vi "setTime.vi"(0 "connection ID":refnum<k5>, 1 "day":i32, 2 "month":i32, 3 "year":i32, 4 "hour":i32, 5 "error":errorcluster, 6 "minute":i32, 7 "second":i32) -> (14 "connection ID out":refnum<k5>, 19 "error out":errorcluster)   [LabVIEW 2016, in "amc_api.lvlib"]
doc: "Sets system time manually."
uses:
  amc_api.lvlib
panel:
  out "jsonRespIn":string
  out "JSON-response":string="{\"jsonrpc\":\"2.0\",\"method\":\"\",\"params\":[5,1.245,true,\"name\"],\"id\":\"1\"}"
  out "JSON request":string
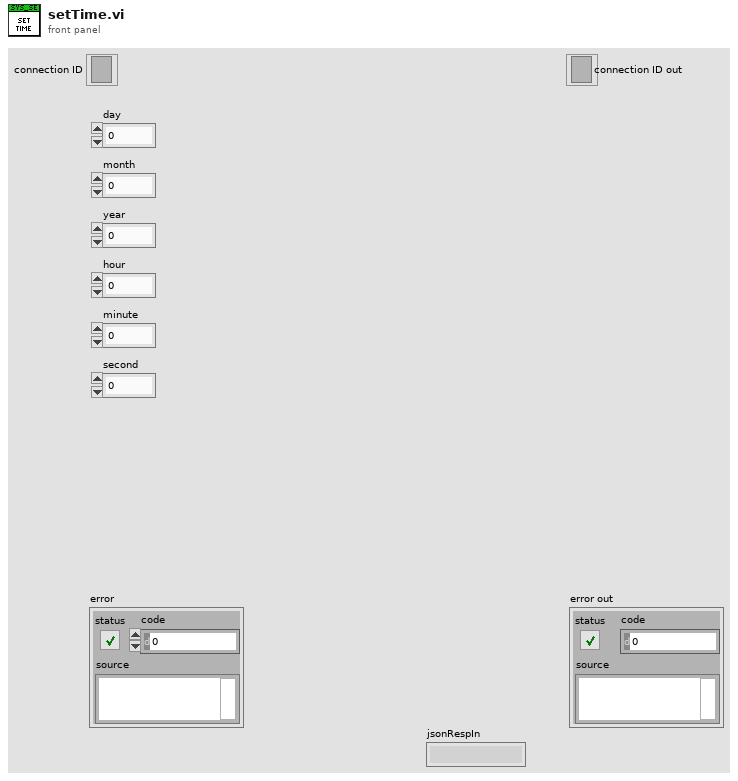
[diagram p1: front panel]
types:
  T1 = cluster{"jsonrpc":string, "method":string, "params":string[], "id":string, "api":i32, "pid":string}
  T2 = enum16{"Standard", "Buffered", "CRLF", "Immediate"}
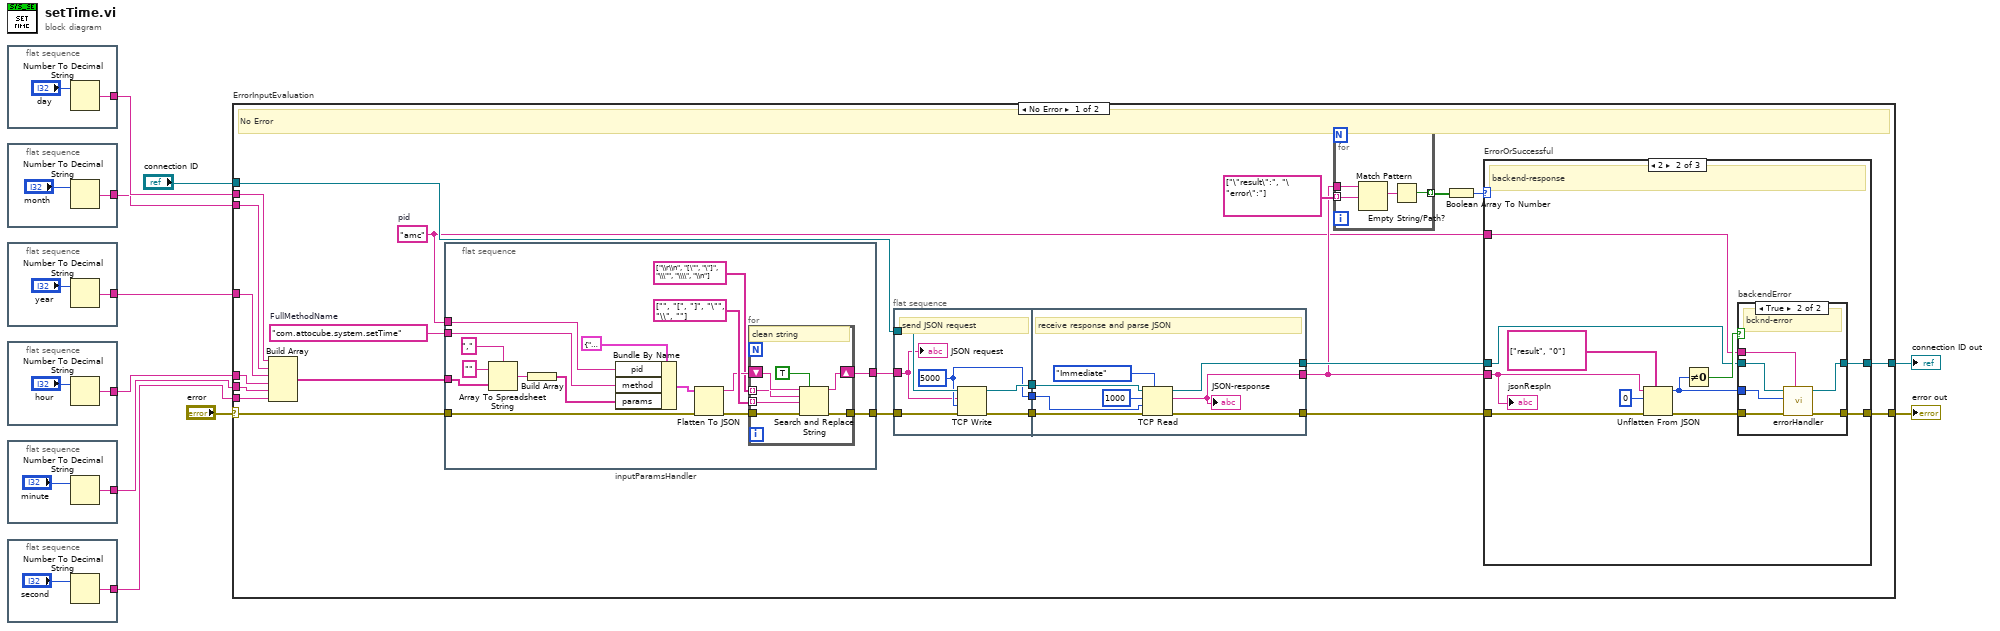
[diagram p0: block diagram]
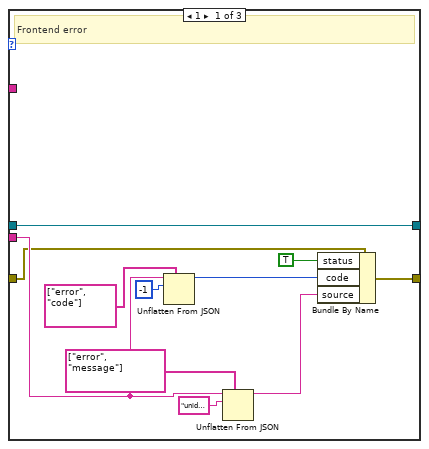
[diagram p2: hidden frame]
diagram:
  n1 = flat-sequence "in_integer" {
    tunnel: [w11] -> w6
    frame #0 {
      n2 = Number To Decimal String(number="day") -> (decimal integer string=w11:string)  [unwired: 1 in]
    }
  }
  n3 = flat-sequence "in_integer" {
    tunnel: [w13] -> w5
    frame #0 {
      n4 = Number To Decimal String(number="month") -> (decimal integer string=w13:string)  [unwired: 1 in]
    }
  }
  n5 = flat-sequence "in_integer" {
    tunnel: [w15] -> w4
    frame #0 {
      n6 = Number To Decimal String(number="year") -> (decimal integer string=w15:string)  [unwired: 1 in]
    }
  }
  n7 = flat-sequence "in_integer" {
    tunnel: [w17] -> w3
    frame #0 {
      n8 = Number To Decimal String(number="hour") -> (decimal integer string=w17:string)  [unwired: 1 in]
    }
  }
  n9 = flat-sequence "in_integer" {
    tunnel: [w19] -> w2
    frame #0 {
      n10 = Number To Decimal String(number="minute") -> (decimal integer string=w19:string)  [unwired: 1 in]
    }
  }
  n11 = flat-sequence "in_integer" {
    tunnel: [w21] -> w1
    frame #0 {
      n12 = Number To Decimal String(number="second") -> (decimal integer string=w21:string)  [unwired: 1 in]
    }
  }
  n13 = case "ErrorInputEvaluation" shown="No Error" "error" {
    selector: "error" -> [w39 w120]
    tunnel: "connection ID" -> [w43 w121]
    tunnel: [w30 w120] -> w9
    tunnel: [w31 w121] -> w8
    tunnel: w6 -> [w28 _]
    tunnel: w5 -> [w27 _]
    tunnel: w4 -> [w26 _]
    tunnel: w3 -> [w25 _]
    tunnel: w2 -> [w24 _]
    tunnel: w1 -> [w23 _]
    frame No Error {
      w29 = "amc"  # pid
      w40 = "com.attocube.system.setTime"  # FullMethodName
      # "No Error"
      n14 = Build Array ("ParametersArrayString")(w28, w27, w26, w25, w24, w23) -> (w38:string[])
      n15 = flat-sequence "inputParamsHandler" {
        tunnel: [w84] -> w37
        tunnel: w38 -> [w90]
        tunnel: w39 -> [w89]
        tunnel: [w86] -> w36
        tunnel: w40 -> [w80]
        tunnel: w29 -> [w79]
        frame #0 {
          n16 = Array To Spreadsheet String(delimiter (Tab)=",", array=w90, 3:"" ("format string")) -> (spreadsheet string=w92:string)
          n17 = Build Array "Build Array"(w92) -> (w81:string[])
          n18 = Bundle By Name(cluster=T1 {"jsonrpc"="2.0", "method"="com.attocube.amc.res.setRESReadOutFreq", "params"=[], "id"="1", "api"=2, "pid"=""} ("Cluster"), "pid"=w79, "method"=w80, "params"=w81) -> (w91:T1)
          n19 = Flatten To JSON(anything=w91, error in (no error)=w89) -> (JSON string=w85:string, 11:w87:errorcluster)  [unwired: 1 in]
          n20 = for {
            tunnel: string[] ["\\r\\n", "[\"", "\"]", "\\\"", "\\\\", "\\n"] ("search string") -> [w98] mode=indexing
            tunnel: string[] ["", "[", "]", "\"", "\\", ""] ("replace string (\"\")") -> [w97] mode=indexing
            shift-right: [w100] -> w84
            shift-left: w85 -> [w99]
            tunnel: w87 -> [w96]
            tunnel: [w95] -> w86
            # "clean string"
            n21 = Search and Replace String(replace all?=TRUE ("replace all? (F)"), input string=w99, search string=w98, replace string=w97, error in=w96) -> (result string=w100:string, error out=w95:errorcluster)  [unwired: 3 in, 2 out]
          }
        }
      }
      n22 = flat-sequence {
        tunnel: w43 -> [w111]
        tunnel: [w109] -> w46
        tunnel: [w110] -> w45
        tunnel: w36 -> [w106]
        tunnel: [w108] -> w44
        tunnel: w37 -> [w107]
        tunnel: [w115] -> w35
        tunnel: w46 -> [w117]
        tunnel: w45 -> [w116]
        tunnel: [w113] -> w34
        tunnel: w44 -> [w114]
        tunnel: [w112] -> w33
        frame #0 {
          w108 = 5000 ("timeout ms (25000)")
          # "send JSON request"
          n23 = TCP Write(connection ID=w111, data in=w107, error in (no error)=w106, 9:w108) -> (connection ID out=w109:refnum<k5>, error out=w110:errorcluster)  [unwired: 1 out]
          "JSON request" <- w107
        }
        frame #1 {
          # "receive response and parse JSON"
          n24 = TCP Read(connection ID=w117, bytes to read=1000, error in (no error)=w116, 7:T2."Immediate" ("mode (standard)"), 9:w114) -> (connection ID out=w115:refnum<k5>, data out=w112:string, error out=w113:errorcluster)
          "JSON-response" <- w112
        }
      }
      n25 = for {
        tunnel: string[] ["\"result\":", "\"error\":"] ("path") -> [w104] mode=indexing
        tunnel: [w102] -> w41 mode=indexing
        tunnel: w33 -> [w105]
        n26 = Match Pattern(string=w105, regular expression=w104) -> (match substring=w103:string)  [unwired: 1 in, 3 out]
        n27 = Empty String/Path?(string/path=w103) -> (empty?=w102:bool)
      }
      n28 = Boolean Array To Number(Boolean array=w41) -> (number=w32:u32)
      n29 = case "ErrorOrSuccessful" shown="2" w32 {
        tunnel: w33 -> [w49 w60 _]
        tunnel: w35 -> [w47 w62 w78]
        tunnel: [w47 w61 w78] -> w31
        tunnel: [w50 w58 w77] -> w30
        tunnel: w34 -> [w48 w59 w77]
        tunnel: w29 -> [_ w63 _]
        frame 1 {
          # "Frontend error"
          n30 = Unflatten From JSON(path=string[] ["error", "code"], JSON string=w49, type and defaults=-1) -> (value=w56:i32)  [unwired: 4 in, 1 out]
          n31 = Unflatten From JSON(path=string[] ["error", "message"], JSON string=w49, type and defaults="unidentified error") -> (value=w57:string)  [unwired: 4 in, 1 out]
          n32 = Bundle By Name(cluster=w48, "status"=TRUE, "code"=w56, "source"=w57) -> (w50:errorcluster)
        }
        frame 2 {
          # "backend-response"
          n33 = Unflatten From JSON(path=string[] ["result", "0"], JSON string=w60, type and defaults=0, error in (no error)=w59) -> (value=w64:i32, error out=w66:errorcluster)  [unwired: 3 in]
          n34 = Not Equal To 0?(x=w64) -> (x != 0?=w65:bool)
          n35 = case "backendError" shown="True" w65 {
            tunnel: w64 -> [_ w76]
            tunnel: w66 -> [w70 w75]
            tunnel: [w69 w74] -> w61
            tunnel: [w70 w73] -> w58
            tunnel: w62 -> [w69 w72]
            tunnel: w63 -> [_ w71]
            frame False {
              # "successful"
            }
            frame True {
              # "bcknd-error"
              n36 = call "errorHandler.vi"("pid"=w71, "error in"=w75, "errNbr"=w76, "connection ID"=w72) -> ("error out 2"=w73:errorcluster, "connection ID out"=w74:refnum<k5>)  [unwired: 6 in]
            }
          }
          "jsonRespIn" <- w60
        }
        frame Default {
          # "NoResponse"
        }
      }
    }
    frame Error {
      # "Error"
    }
  }
  "error out" <- w9
  "connection ID out" <- w8
